vi "Write Dwell Time.vi"(8 "error in (no error)":errorcluster, 10 "Dwell Time":dbl[unit], 11 "Reader.lvclass in":refnum<class "Reader.lvclass">) -> (0 "error out":errorcluster, 3 "Reader.lvclass out":refnum<class "Reader.lvclass">)   [LabVIEW 2009, in "Reader.lvclass"]
uses:
  Reader.lvclass
  Reader.lvclass/Reader.ctl
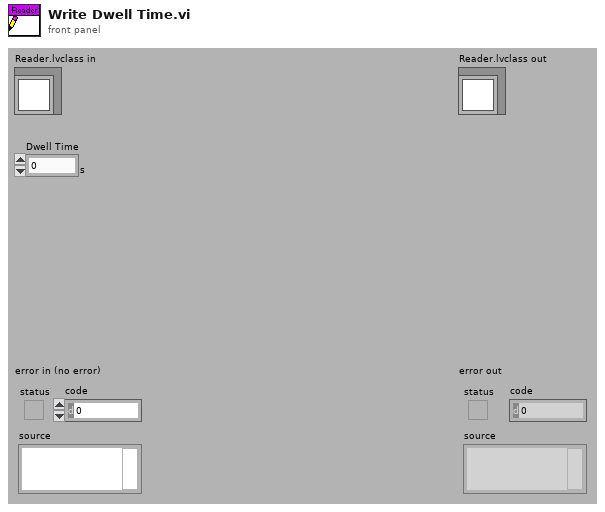
[diagram p1: front panel]
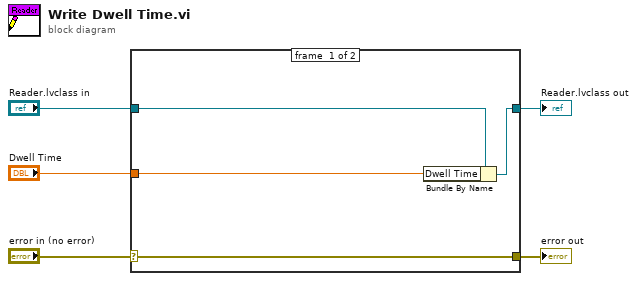
[diagram p0: block diagram]
diagram:
  n1 = case shown="No Error" "error in (no error)" {
    selector: "error in (no error)" -> [w9 w10]
    tunnel: [w9 w10] -> w4
    tunnel: [w7 w11] -> w2
    tunnel: "Reader.lvclass in" -> [w8 w11]
    tunnel: "Dwell Time" -> [w6 _]
    frame #0 {
      n2 = Bundle By Name(cluster=w8, "Dwell Time"=w6) -> (w7:refnum<class "Reader.lvclass">)
    }
    frame #1 {
    }
  }
  "error out" <- w4
  "Reader.lvclass out" <- w2
